vi "QTMDriver.vi"(0 "connection ID":refnum<k5>, 1 "Ring":T1, 5 "DataIn":dbl[](array[numeric]), 7 "QTMqueue":refnum<queue>, 9 "VI Refnum QTMTask":refnum<vi>, 11 "error in":errorcluster, 12 "timeout ms (25000)":i32=6000, 13 "DataOutIndex":i32=1) -> (3 "ArrayOut":dbl[](array[numeric]), 4 "connection ID out":refnum<k5>, 6 "DataOut":dbl[](array[numeric]), 8 "QTMqueue Out":refnum<queue>, 10 "return count":u32, 14 "VI Refnum QTMTask Out":refnum<vi>, 15 "error out":errorcluster)   [LabVIEW 2014]
uses:
  CustomIO.ctl
  <vilib>/Instr/_visa.llb/VISA Configure Serial Port (Instr).vi
panel:
  in  "flow control":u32(ring) items=["None", "XON/XOFF", "RTS/CTS", "XON/XOFF & RTS/CTS", "DTR/DSR", "XON/XOFF & DTR/DSR"]
  in  "stop bits":u32(ring)=10 items=["1.0"=10, "1.5"=15, "2.0"=20]
  in  "parity":enum32{"None", "Odd", "Even", "Mark", "Space"}(ring)=enum."Even"
  in  "data bits":u32=8
  in  "baud rate":u32=115200
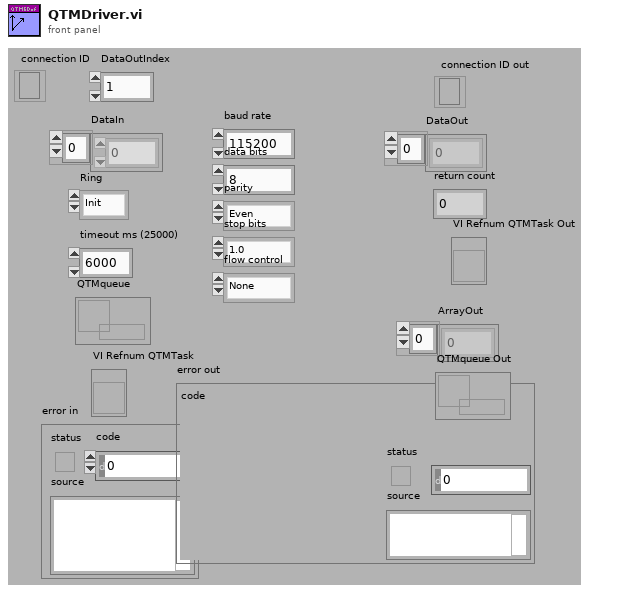
[diagram p1: front panel]
types:
  T1 = typedef "CustomIO.ctl" = enum16{"Init", "Read", "Write", "Close", "N/O"}
  T2 = enum16{"big-endian, network order", "native, host order", "little-endian"}
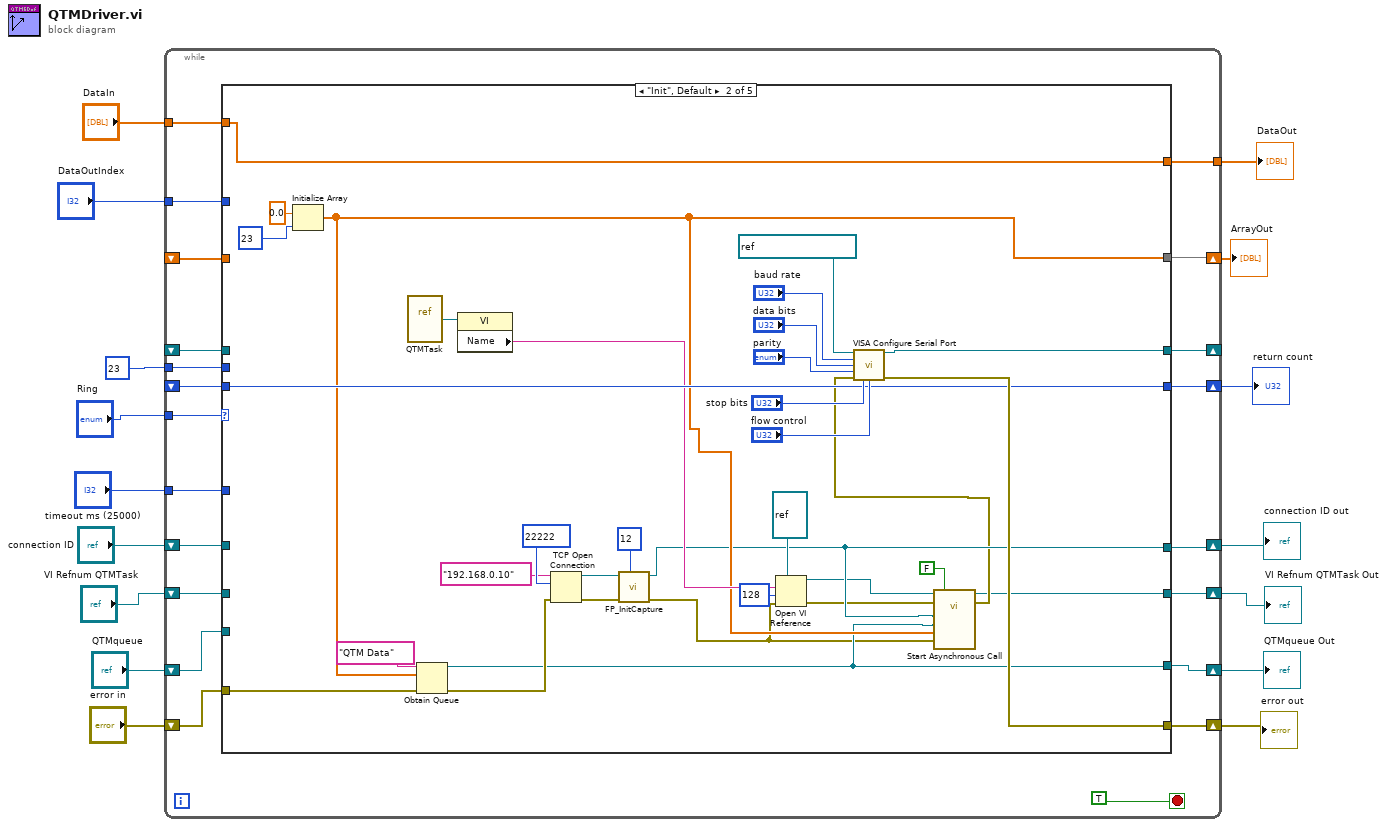
[diagram p0: block diagram]
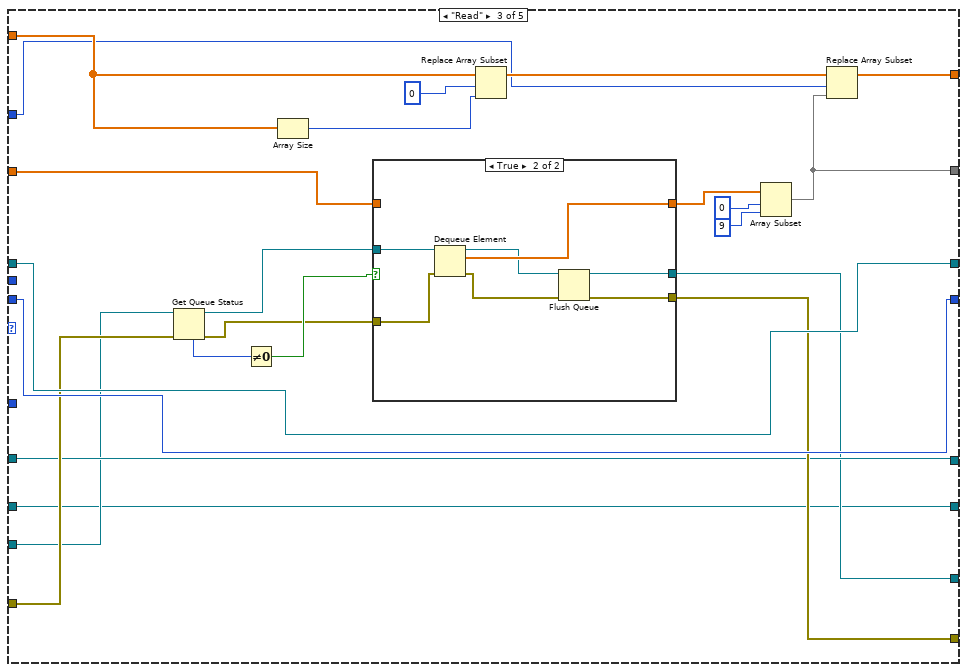
[diagram p3: hidden frame]
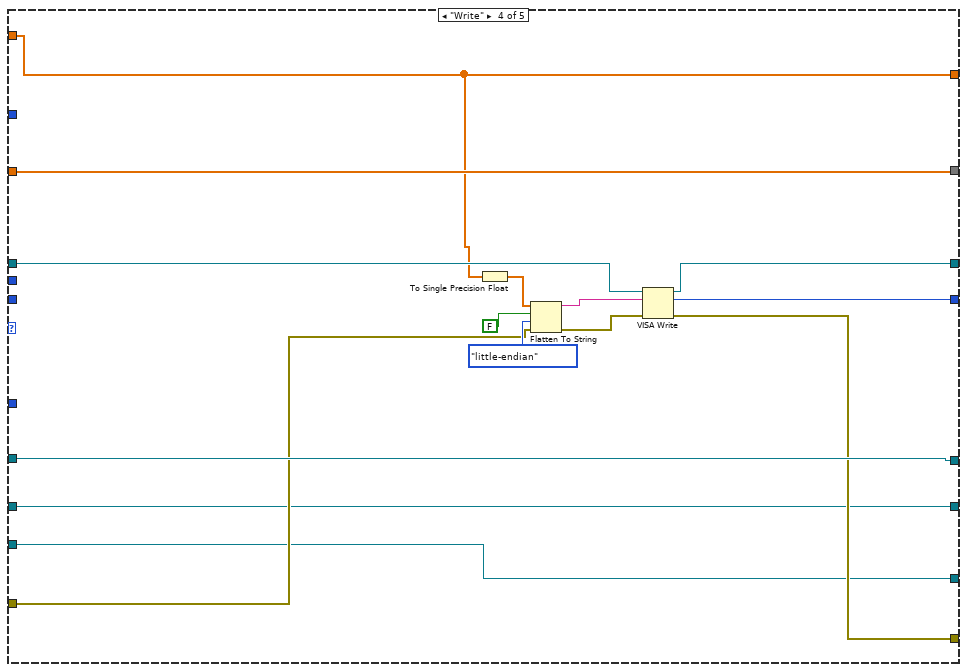
[diagram p5: hidden frame]
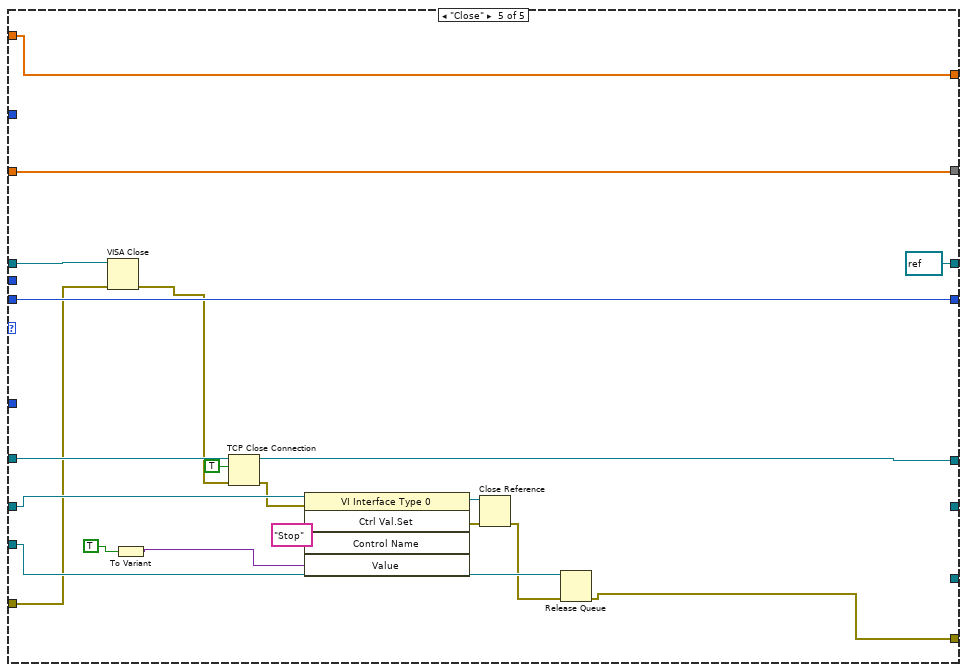
[diagram p6: hidden frame]
diagram:
  n1 = while {
    tunnel: "Ring" -> [w37]
    shift-right: [w36] -> w6
    shift-left: _ -> [w35]
    tunnel: 23 -> [w34]
    shift-right: [w32] -> w14
    shift-left: "error in" -> [w33]
    shift-right: [w30] -> w12
    shift-left: "connection ID" -> [w31]
    tunnel: "DataIn" -> [w29]
    tunnel: [w28] -> w10
    tunnel: "DataOutIndex" -> [w27]
    tunnel: "timeout ms (25000)" -> [w26]
    shift-right: [w25] -> _
    shift-left: _ -> [w24]
    shift-right: [w23] -> w7
    shift-left: _ -> [w22]
    shift-right: [w21] -> w3
    shift-left: "QTMqueue" -> [w20]
    shift-right: [w19] -> w1
    shift-left: "VI Refnum QTMTask" -> [w18]
    stop <- TRUE stop-if-true
    n2 = case shown="\"Init\", Default" w37 {
      tunnel: [w45 w54 w79 w120 w143] -> w36
      tunnel: w35 -> [w45 _ w90 w120 w143]
      tunnel: w34 -> [_ _ _ _ _]
      tunnel: w33 -> [w44 w60 w93 w117 w135]
      tunnel: [w44 w65 w87 w116 w134] -> w32
      tunnel: w31 -> [w38 _ w86 w126 w145]
      tunnel: [w38 w52 w86 w126 w144] -> w30
      tunnel: w29 -> [w43 w74 w98 w114 w142]
      tunnel: [w43 w74 w97 w114 w142] -> w28
      tunnel: w27 -> [_ _ w96 _ _]
      tunnel: w26 -> [_ _ _ _ _]
      tunnel: [w42 w66 w95 w118 refnum<visa-resource-name> refnum ("VISA resource name out")] -> w25
      tunnel: w24 -> [w42 _ w95 w119 w141]
      tunnel: [w41 w64 w94 w115 w139] -> w23
      tunnel: w22 -> [w41 w64 w94 _ w139]
      tunnel: [w40 w53 w84 w113 _] -> w21
      tunnel: w20 -> [w40 _ w85 w113 w137]
      tunnel: [w39 w50 w83 w112 _] -> w19
      tunnel: w18 -> [w39 _ w83 w112 w138]
      frame "N/O" {
      }
      frame "Init", Default {
        n3 = Initialize Array(0.0 ("element"), 23) -> (w54:dbl[])
        n4 = vi-ref "QTMTask.vi"() -> (w55:refnum<vi>)
        n5 = Obtain Queue(name (unnamed)="QTM Data", element data type=w54, error in (no error)=w60) -> (queue out=w53:refnum<queue>, error out=w59:errorcluster)  [unwired: 2 in, 1 out]
        n6 = property class="VI"(reference=w55) -> ("Name"=w57:string)  [unwired: 1 in, 2 out]
        n7 = TCP Open Connection(address="192.168.0.10", remote port or service name=u16 22222, error in (no error)=w59) -> (connection ID=w78:refnum<k5>, error out=w77:errorcluster)  [unwired: 2 in]
        n8 = call "FP_InitCapture.vi"("ComponentType"=u32 12, "error out 2"=w77, "connection ID"=w78) -> ("error out"=w46:errorcluster, "connection ID out"=w52:refnum<k5>)  [unwired: 5 in, 2 out]
        n9 = Open VI Reference(type specifier VI Refnum (for type only)=refnum<vi> refnum, vi path=w57, options=128, error in (no error)=w46) -> (vi reference=w48:refnum<vi>, error out=w47:errorcluster)  [unwired: 2 in]
        n10 = call-by-ref "Start Asynchronous Call"(reference=w48, error in=w47, "Stop"=FALSE, "error in"=w46, "ArrayIn"=w54, "QTMqueue"=w53, "connection ID"=w52) -> (reference out=w50:refnum<vi>, error out=w51:errorcluster)  [unwired: 4 in, 2 out]
        n11 = call-poly "VISA Configure Serial Port"("VISA resource name"=refnum<visa-resource-name> "ASRL1::INSTR", "baud rate (9600)"="baud rate", "data bits (8)"="data bits", "parity (0:none)"="parity", "error in (no error)"=w51, "stop bits (10: 1 bit)"="stop bits", "flow control (0:none)"="flow control") -> ("VISA resource name out"=w66:refnum<visa-resource-name>, "error out"=w65:errorcluster)  [unwired: 7 out]
      }
      frame "Read" {
        n12 = Get Queue Status(queue=w85, error in (no error)=w93) -> (queue out=w89:refnum<queue>, error out=w88:errorcluster, # elements in queue=w92:i32)  [unwired: 1 in, 5 out]
        n13 = Not Equal To 0?(x=w92) -> (x != 0?=w91:bool)
        n14 = Array Size(array=w98) -> (size(s)=w99:i32)
        n15 = case shown="True" w91 {
          tunnel: w90 -> [w104 _]
          tunnel: w89 -> [w102 w111]
          tunnel: [w104 w110] -> w80
          tunnel: w88 -> [w103 w107]
          tunnel: [w103 w106] -> w87
          tunnel: [w102 w105] -> w84
          frame False {
          }
          frame True {
            n16 = Dequeue Element(queue=w111, error in (no error)=w107) -> (queue out=w109:refnum<queue>, element=w110:dbl[], error out=w108:errorcluster)  [unwired: 1 in, 1 out]
            n17 = Flush Queue(queue=w109, error in (no error)=w108) -> (queue out=w105:refnum<queue>, error out=w106:errorcluster)  [unwired: 1 out]
          }
        }
        n18 = Replace Array Subset(array=w98, new element=w99, index=0) -> (w100:dbl[])
        n19 = Array Subset(array=w80, index=0, length=9) -> (w79:dbl[])
        n20 = Replace Array Subset(array=w100, new element=w79, index=w96) -> (w97:dbl[])
      }
      frame "Write" {
        n21 = To Single Precision Float(number=w114) -> (single precision float=w122:sgl[])
        n22 = Flatten To String(anything=w122, prepend array or string size? (T)=FALSE, byte order (0:big-endian, network order)=T2."little-endian", error in (no error)=w117) -> (data string=w121:string, error out=w123:errorcluster)  [unwired: 1 out]
        n23 = VISA Write(VISA resource name=w119, write buffer=w121, error in (no error)=w123) -> (VISA resource name out=w118:refnum<visa-resource-name>, return count=w115:u32, error out=w116:errorcluster)
      }
      frame "Close" {
        n24 = VISA Close(VISA resource name=w141, error in (no error)=w135) -> ()  [unwired: 1 out]
        n25 = To Variant(anything=TRUE) -> (Variant=w130:variant)
        n26 = TCP Close Connection(connection ID=w145, abort (F)=TRUE, error in (no error)=w135) -> (connection ID out=w144:refnum<k5>, error out=w128:errorcluster)
        n27 = invoke class="VI Interface Type 0" method="Ctrl Val.Set"(reference=w138, error in=w128, "Control Name"="Stop", "Value"=w130) -> (reference out=w133:refnum<vi>, error out=w127:errorcluster)  [unwired: 1 in, 3 out]
        n28 = Close Reference(reference=w133, error in (no error)=w127) -> (error out=w136:errorcluster)
        n29 = Release Queue(queue=w137, error in (no error)=w136) -> (error out=w134:errorcluster)  [unwired: 1 in, 2 out]
      }
    }
  }
  "error out" <- w14
  "connection ID out" <- w12
  "DataOut" <- w10
  "return count" <- w7
  "ArrayOut" <- w6
  "QTMqueue Out" <- w3
  "VI Refnum QTMTask Out" <- w1
